vi "信息插入.vi"() -> ()   [LabVIEW 2018]
uses:
  <vilib>/addons/database/Connection.llb/DB Tools Open Connec (Path).vi
  <vilib>/addons/database/NI_Database_API.lvlib
panel:
  out "columns":string[](array[string])
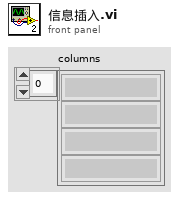
[diagram p1: front panel]
types:
  T1 = typedef "NI_Database_API.lvlib/Conn ObjectReference.ctl" = refnum<k1>
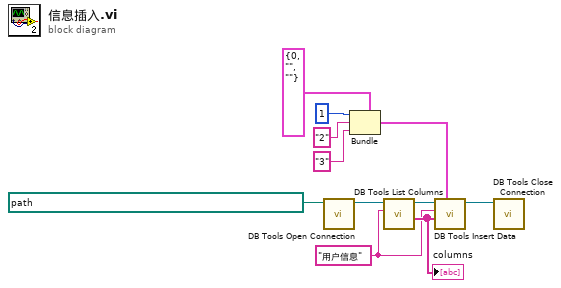
[diagram p0: block diagram]
diagram:
  w7 = "用户信息" ("table")
  n1 = call-poly <vilib>:"DB Tools Open Connection.vi"("connection information"=path "D:/SoftwareWS/LabVIEW/LV-DB/file/用户信息.udl") -> ("connection reference"=w10:T1)  [unwired: 7 in, 1 out]
  n2 = Bundle(cluster=cluster{i32, string, string} {0, "", ""}, 1, "2", "3") -> (w5:cluster{i32, string, string})
  n3 = call <vilib>:"DB Tools List Columns.vi"("table"=w7, "connection reference"=w10) -> ("columns"=w8:string[], "connection reference out"=w9:T1)  [unwired: 2 in, 2 out]
  "columns" <- w8
  n4 = call <vilib>:"DB Tools Insert Data.vi"("data"=w5, "columns"=w8, "table"=w7, "connection reference"=w9) -> ("connection reference out"=w6:T1)  [unwired: 6 in, 1 out]
  n5 = call <vilib>:"DB Tools Close Connection.vi"("connection reference"=w6) -> ()  [unwired: 6 in, 1 out]
